vi "X_AxisMotorControlSetupAndHome.vi"(11 "Automation Refnum in":refnum<k7>(container)) -> (2 "X Translation Serial Number":i32=40849496, 3 "Automation Refnum out":refnum<k7>)   [LabVIEW 2020]
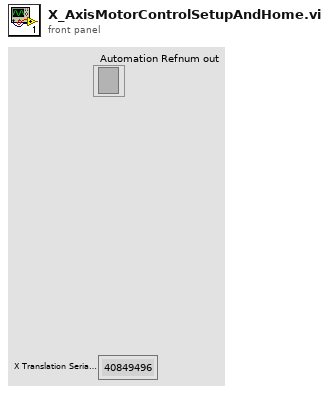
[diagram p1: front panel]
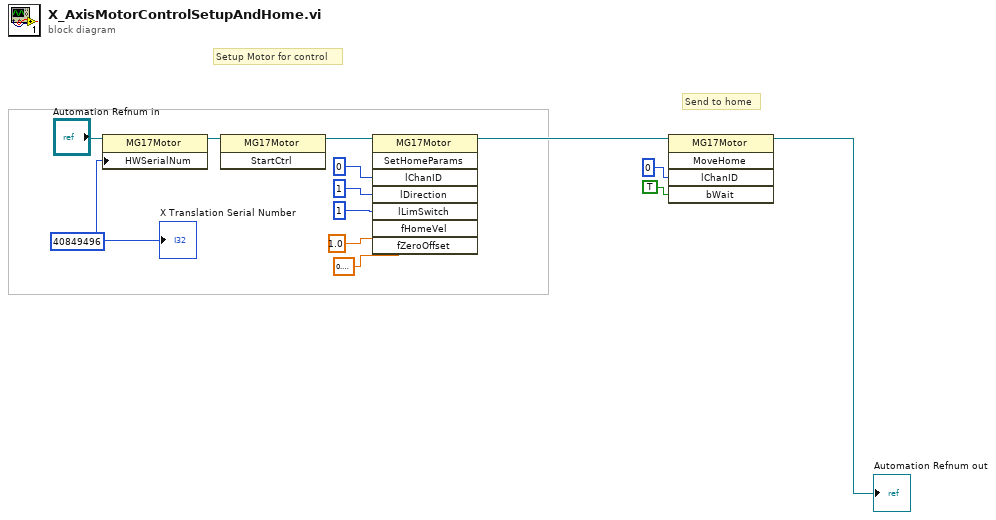
[diagram p0: block diagram]
diagram:
  w12 = 40849496 ("Serial Number")
  # "Setup Motor for control"
  # "Send to home"
  n1 = property on="Property Node" class="MG17Motor"(reference="Automation Refnum in", "HWSerialNum"=w12) -> (reference out=w4:refnum<k7>)  [unwired: 1 in, 1 out]
  n2 = invoke class="MG17Motor" method="StartCtrl"(reference=w4) -> (reference out=w2:refnum<k7>)  [unwired: 2 in, 2 out]
  n3 = invoke class="MG17Motor" method="SetHomeParams"(reference=w2, "lChanID"=0, "lDirection"=1, "lLimSwitch"=1, "fHomeVel"=sgl 1.0, "fZeroOffset"=sgl 0.1) -> (reference out=w1:refnum<k7>)  [unwired: 2 in, 7 out]
  n4 = invoke class="MG17Motor" method="MoveHome"(reference=w1, "lChanID"=0, "bWait"=TRUE) -> (reference out=→"Automation Refnum out":refnum<k7>)  [unwired: 2 in, 4 out]
  "X Translation Serial Number" <- w12
